vi "ReadOutput.vi"(8 "error in (no error)":errorcluster, 11 "DAQ_QPT_Throlab in":refnum<class "DAQ_QPD_Throlab.lvclass">) -> (0 "error out":errorcluster, 2 "Output Values":dbl[](array[numeric]), 3 "DAQ_QPT_Throlab out":refnum<class "DAQ_QPD_Throlab.lvclass">)   [LabVIEW 2020, in "DAQ_QPD_Throlab.lvlib" / "DAQ_QPD_Throlab.lvclass"]
uses:
  DAQ_QPD_Throlab.lvclass
  DAQ_QPD_Throlab.lvclass/DAQ_QPD_Throlab.ctl
  Hardware Abstraction Layer/Component/DAQ/DAQ/DAQ.lvclass
  Dependency/TIRF-Lock.dll
panel:
  in  "Display":bool=TRUE
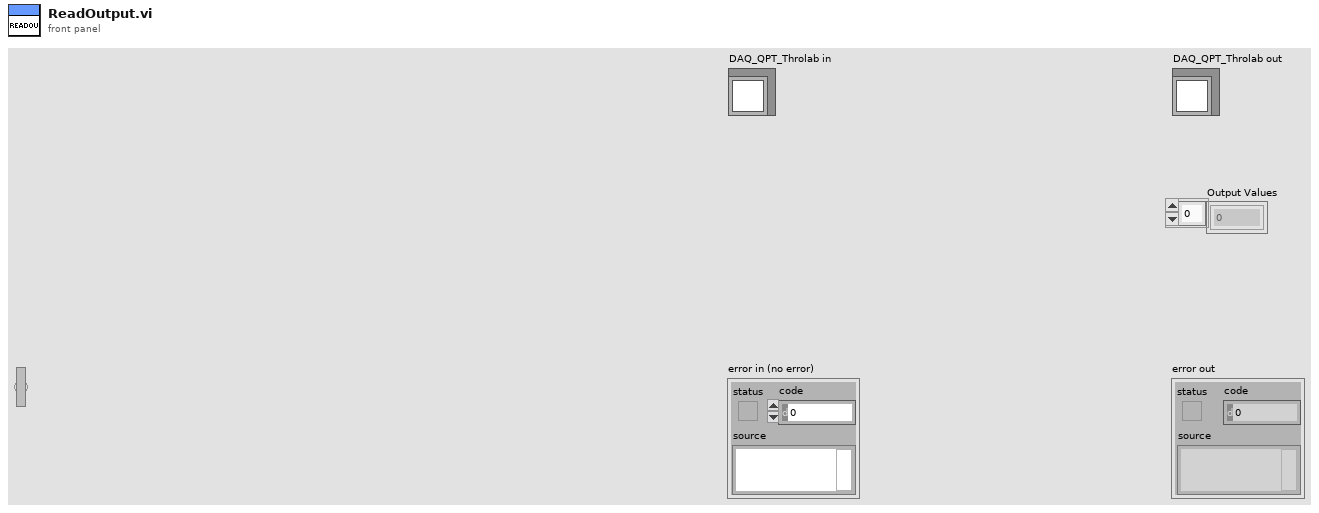
[diagram p1: front panel]
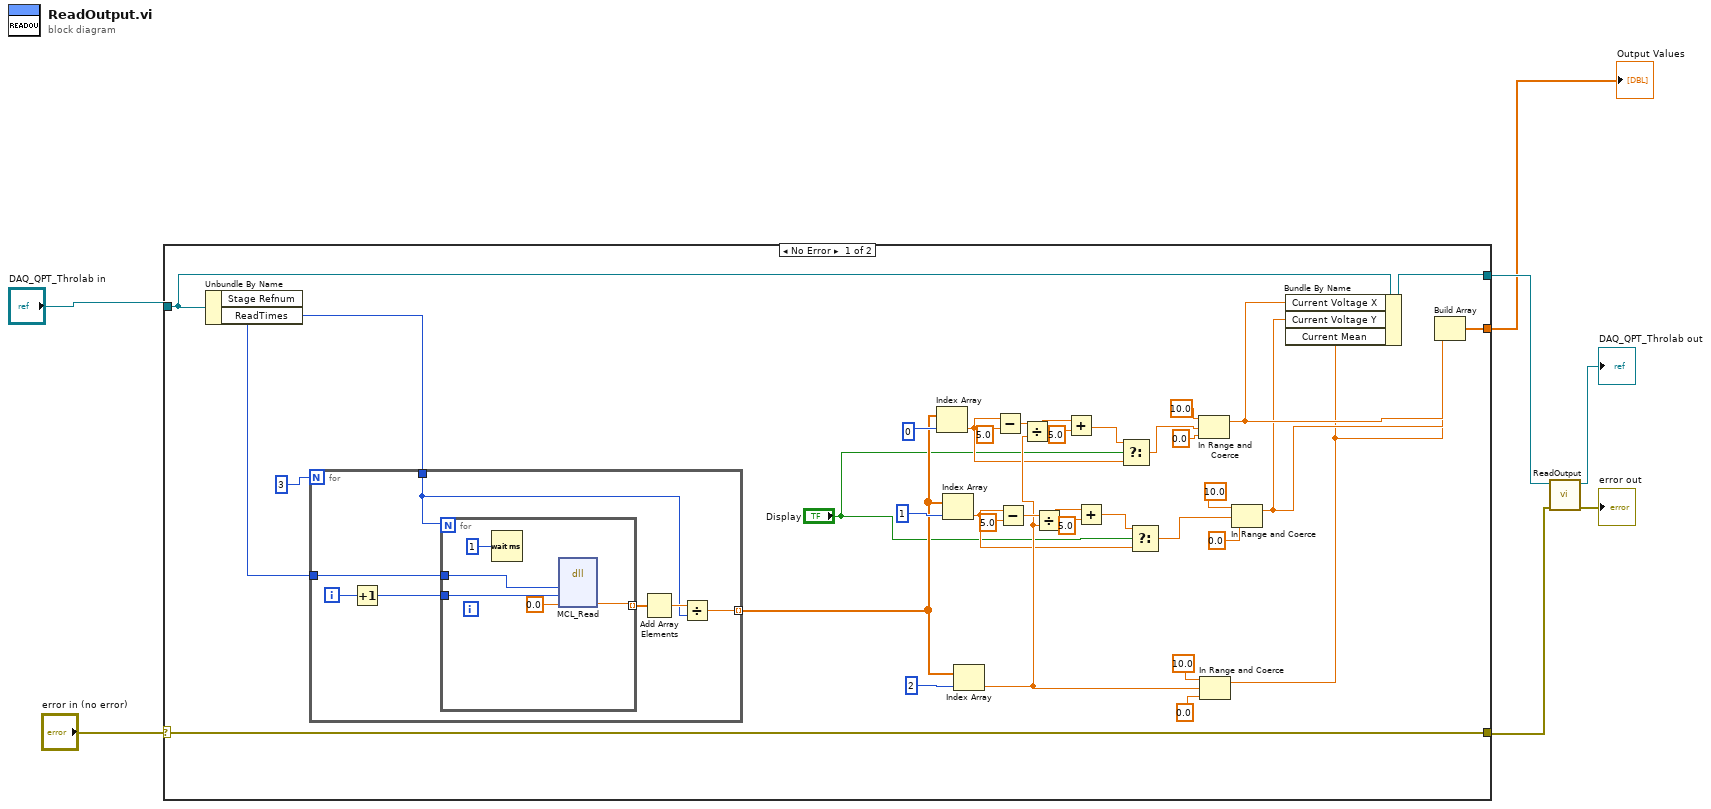
[diagram p0: block diagram]
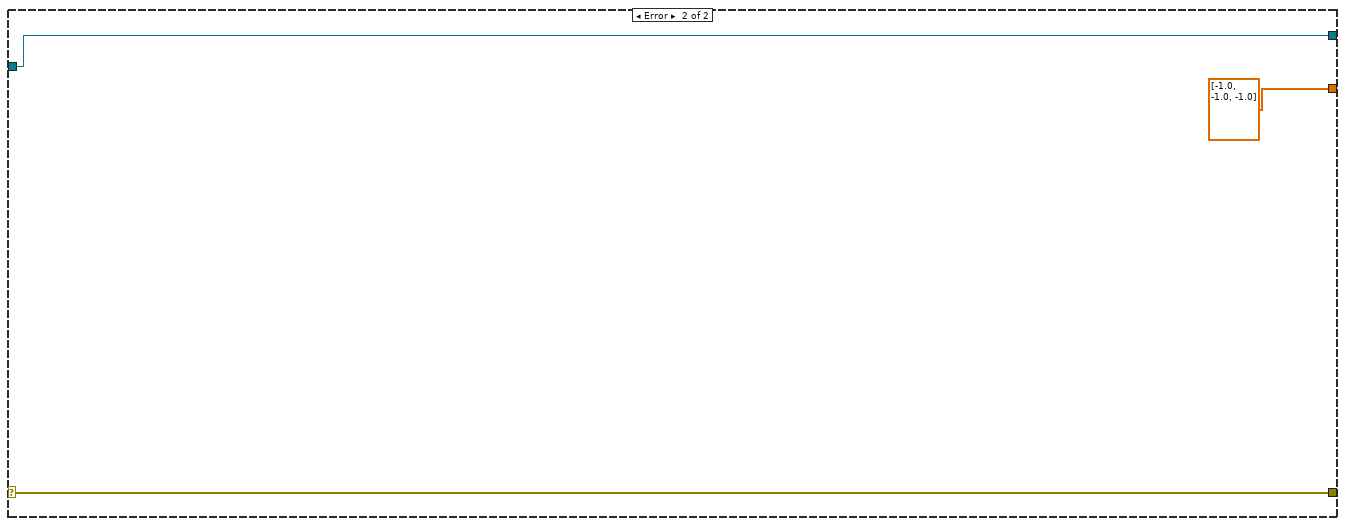
[diagram p2: hidden frame]
diagram:
  n1 = case shown="No Error" "error in (no error)" {
    selector: "error in (no error)" -> [w16 w58]
    tunnel: [w16 w58] -> w4
    tunnel: "DAQ_QPT_Throlab in" -> [w12 w56]
    tunnel: [w14 dbl[] [-1.0, -1.0, -1.0]] -> w1
    tunnel: [w11 w56] -> w2
    frame No Error {
      n2 = Unbundle By Name(w12) -> ("Stage Refnum"=w15:i32, "ReadTimes"=w13:i32)
      n3 = for {
        N: 3 -> [_]
        tunnel: [w49] -> w27 mode=indexing
        tunnel: w15 -> [w46]
        tunnel: w13 -> [w45]
        i -> [w47]
        n4 = Increment(x=w47) -> (x+1=w48:i32)
        n5 = for {
          N: w45 -> [_]
          tunnel: w46 -> [w53]
          tunnel: w48 -> [w54]
          tunnel: [w51] -> w44 mode=indexing
          n6 = Wait (ms)(milliseconds to wait=1) -> ()  [unwired: 1 out]
          n7 = dll-call lib="D:/Daguan/Development/MMicroscopyFramework/Model/Hardware Layer/Real Hardware/DAQ_QPT_Throlab/DAQ_QPT_Throlab/Dependency/TIRF-Lock.dll" fn="MCL_Read" label="tirf read"("handle"=w53, "axis"=w54, "readValue"=0.0) -> ("readValue"=w51:dbl)  [unwired: 5 in, 3 out]
        }
        n8 = Add Array Elements(numeric array=w44) -> (sum=w50:dbl)
        n9 = Divide(x=w50, y=w45) -> (x/y=w49:dbl)
      }
      n10 = Index Array(array=w27, index=0) -> (element=w21:dbl)
      n11 = Index Array(array=w27, index=1) -> (element=w18:dbl)
      n12 = Index Array(array=w27, index=2) -> (element=w25:dbl)
      n13 = Subtract(x=w21, y=5.0) -> (x-y=w42:dbl)
      n14 = Subtract(x=w18, y=5.0) -> (x-y=w35:dbl)
      n15 = Divide(x=w42, y=w25) -> (x/y=w39:dbl)
      n16 = Divide(x=w35, y=w25) -> (x/y=w33:dbl)
      n17 = Add(x=w39, y=5.0) -> (x+y=w23:dbl)
      n18 = Add(x=w33, y=5.0) -> (x+y=w20:dbl)
      n19 = Select(t=w23, s="Display", f=w21) -> (s? t:f=w22:dbl)
      n20 = Select(t=w20, s="Display", f=w18) -> (s? t:f=w19:dbl)
      n21 = In Range and Coerce(upper limit=10.0, x=w22, lower limit=0.0) -> (coerced(x)=w10:dbl)  [unwired: 1 out]
      n22 = In Range and Coerce(upper limit=10.0, x=w25, lower limit=0.0) -> (coerced(x)=w8:dbl)  [unwired: 1 out]
      n23 = In Range and Coerce(upper limit=10.0, x=w19, lower limit=0.0) -> (coerced(x)=w9:dbl)  [unwired: 1 out]
      n24 = Bundle By Name(cluster=w12, "Current Voltage X"=w10, "Current Voltage Y"=w9, "Current Mean"=w8) -> (w11:refnum<class "DAQ_QPD_Throlab.lvclass">)
      n25 = Build Array(w10, w9, w8) -> (w14:dbl[])
    }
    frame Error {
    }
  }
  "Output Values" <- w1
  n26 = call-parent "ReadOutput.vi"("error in (no error)"=w4, "DAQ in"=w2) -> ("error out"=→"error out":errorcluster, "DAQ out"=→"DAQ_QPT_Throlab out":refnum<class "DAQ_QPD_Throlab.lvclass">)  [unwired: 7 in, 1 out]
